vi "Deploy.vi"(6 "VI reference (current VI)":refnum<vi>, 8 "error in (no error)":errorcluster, 9 "Network Settings in":T3, 10 "Targets in":T4 {"Filtered Targets"."IP Mode" items=["Static"=1, "DHCP/Link-Local"=2, "Link-Local Only"=4, "DHCP Only"=8]}, 11 "Ctl Refs in":T7) -> (0 "error out":errorcluster, 1 "Network Settings out":T3, 2 "Targets out":T4 {"Filtered Targets"."IP Mode" items=["Static"=1, "DHCP/Link-Local"=2, "Link-Local Only"=4, "DHCP Only"=8]}, 3 "Ctl Refs out":T7, 4 "Button State":T2, 5 "Execution State":T1)   [LabVIEW 2013]
uses:
  Controls/Refs.ctl
  Controls/Button Refs.ctl
  Controls/Tab Ctl Refs.ctl
  types/TabStateType.ctl
  Controls/Indicator Refs.ctl
  Controls/Slider Refs.ctl
  Controls/Control Refs.ctl
  Controls/Targets.ctl
  Controls/Detected.ctl
  types/MAX Sys Cfg Target Information.ctl
  Controls/Network Settings.ctl
  types/ButtonStateType.ctl
  types/ExecutionStateType.ctl
  globals/Globals.vi
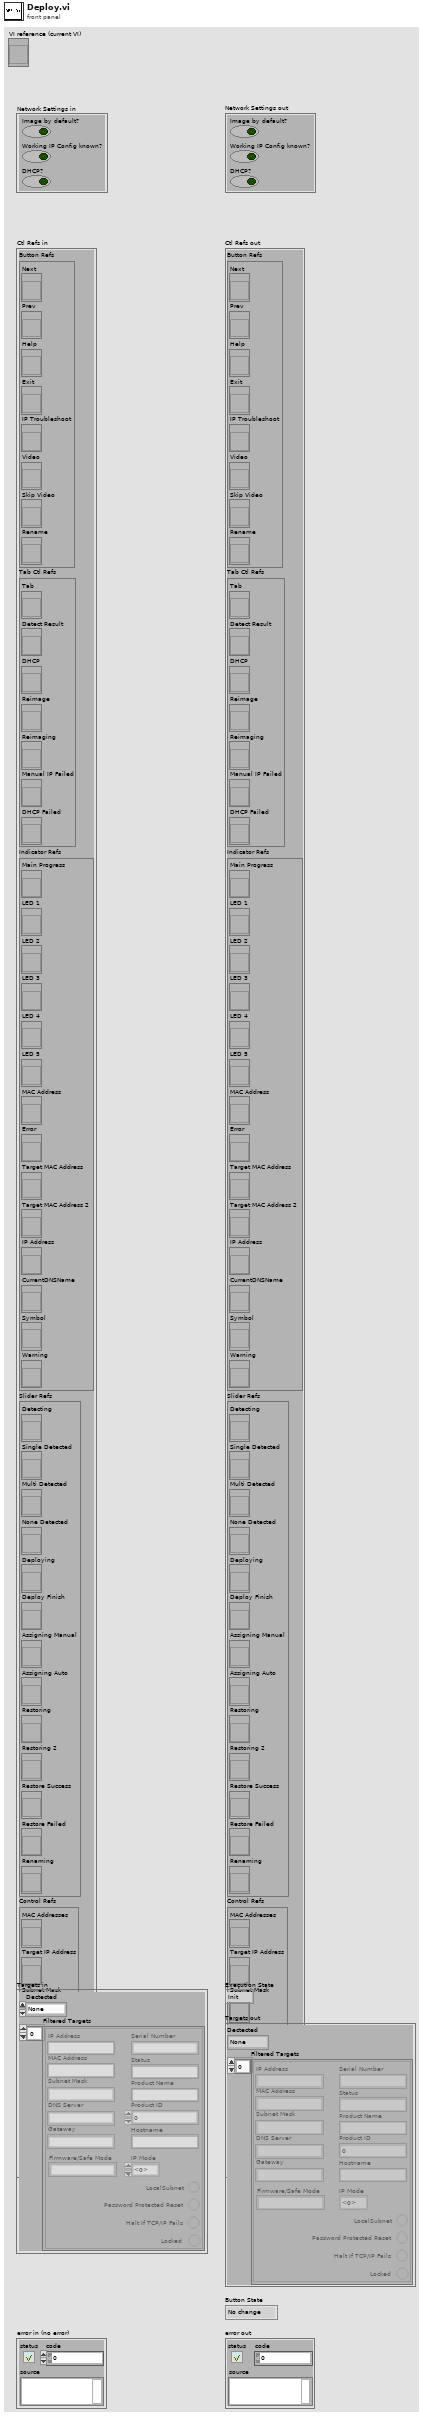
[diagram p1: front panel]
types:
  T1 = typedef "ExecutionStateType.ctl" = enum16{"Init", "Welcome", "Idle", "Detect", "Run Detection", "Detect Fail", "Detect One", "Detect Mult", "Deploy", "DHCP", "Static IP", "Run Deployment", "Connect Verify", "Exit", "Video Wait", "Success", "Troubleshoot", "Troubleshoot 2", "RenameDNS"}
  T2 = typedef "ButtonStateType.ctl" = enum16{"No change", "No Next", "No Prev", "All Disabled", "All Enabled", "Exit Only"}
  T3 = typedef "Network Settings.ctl" = cluster{"Image by default?":bool, "Working IP Config known?":bool, "DHCP?":bool}
  T4 = typedef "Targets.ctl" = cluster{"Dectected":T5, "Filtered Targets":T6[]}
  T5 = typedef "Detected.ctl" = enum16{"None", "Failed", "Single", "Multi"}
  T6 = typedef "MAX Sys Cfg Target Information.ctl" = cluster{"MAC Address":string, "IP Address":string, "Status":string, "Product Name":string, "Hostname":string, "Firmware/Safe Mode":string, "Subnet Mask":string, "Gateway":string, "DNS Server":string, "Serial Number":string, "Product ID":u32, "Locked ":bool, "LocalSubnet":bool, "Halt If TCP/IP Fails":bool, "Password Protected Reset":bool, "IP Mode":i32}
  T7 = typedef "Refs.ctl" = cluster{"Button Refs":T8, "Tab Ctl Refs":T9, "Indicator Refs":T10, "Slider Refs":T11, "Control Refs":T12, "Deploy Message":refnum<vi>}
  T8 = typedef "Button Refs.ctl" = cluster{"Next":refnum<vi>, "Prev":refnum<vi>, "Help":refnum<vi>, "Exit":refnum<vi>, "IP Troubleshoot":refnum<vi>, "Video":refnum<vi>, "Skip Video":refnum<vi>, "Rename":refnum<vi>}
  T9 = typedef "Tab Ctl Refs.ctl" = cluster{"Tab":refnum<vi>, "Detect Result":refnum<vi>, "DHCP":refnum<vi>, "Reimage":refnum<vi>, "Reimaging":refnum<vi>, "Manual IP Failed":refnum<vi>, "DHCP Failed":refnum<vi>}
  T10 = typedef "Indicator Refs.ctl" = cluster{"Main Progress":refnum<vi>, "LED 1":refnum<vi>, "LED 2":refnum<vi>, "LED 3":refnum<vi>, "LED 4":refnum<vi>, "LED 5":refnum<vi>, "MAC Address":refnum<vi>, "Error":refnum<vi>, "Target MAC Address":refnum<vi>, "Target MAC Address 2":refnum<vi>, "IP Address":refnum<vi>, "CurrentDNSName":refnum<vi>, "Symbol":refnum<vi>, "Warning":refnum<vi>}
  T11 = typedef "Slider Refs.ctl" = cluster{"Detecting":refnum<vi>, "Single Detected":refnum<vi>, "Multi Detected":refnum<vi>, "None Detected":refnum<vi>, "Deploying":refnum<vi>, "Deploy Finish":refnum<vi>, "Assigning Manual":refnum<vi>, "Assigning Auto":refnum<vi>, "Restoring":refnum<vi>, "Restoring 2":refnum<vi>, "Restore Success":refnum<vi>, "Restore Failed":refnum<vi>, "Renaming":refnum<vi>}
  T12 = typedef "Control Refs.ctl" = cluster{"MAC Addresses":refnum<vi>, "Target IP Address":refnum<vi>, "Subnet Mask":refnum<vi>, "DNS IP":refnum<vi>, "Default Gateway":refnum<vi>, "DNSName":refnum<vi>}
  T13 = enum32{"Welcome", "Instructions", "Detect", "Run Detection", "Detect Result", "Deploy", "Run Deployment", "Connect Verify", "Success", "DHCP", "Troubleshoot", "System Restore"}
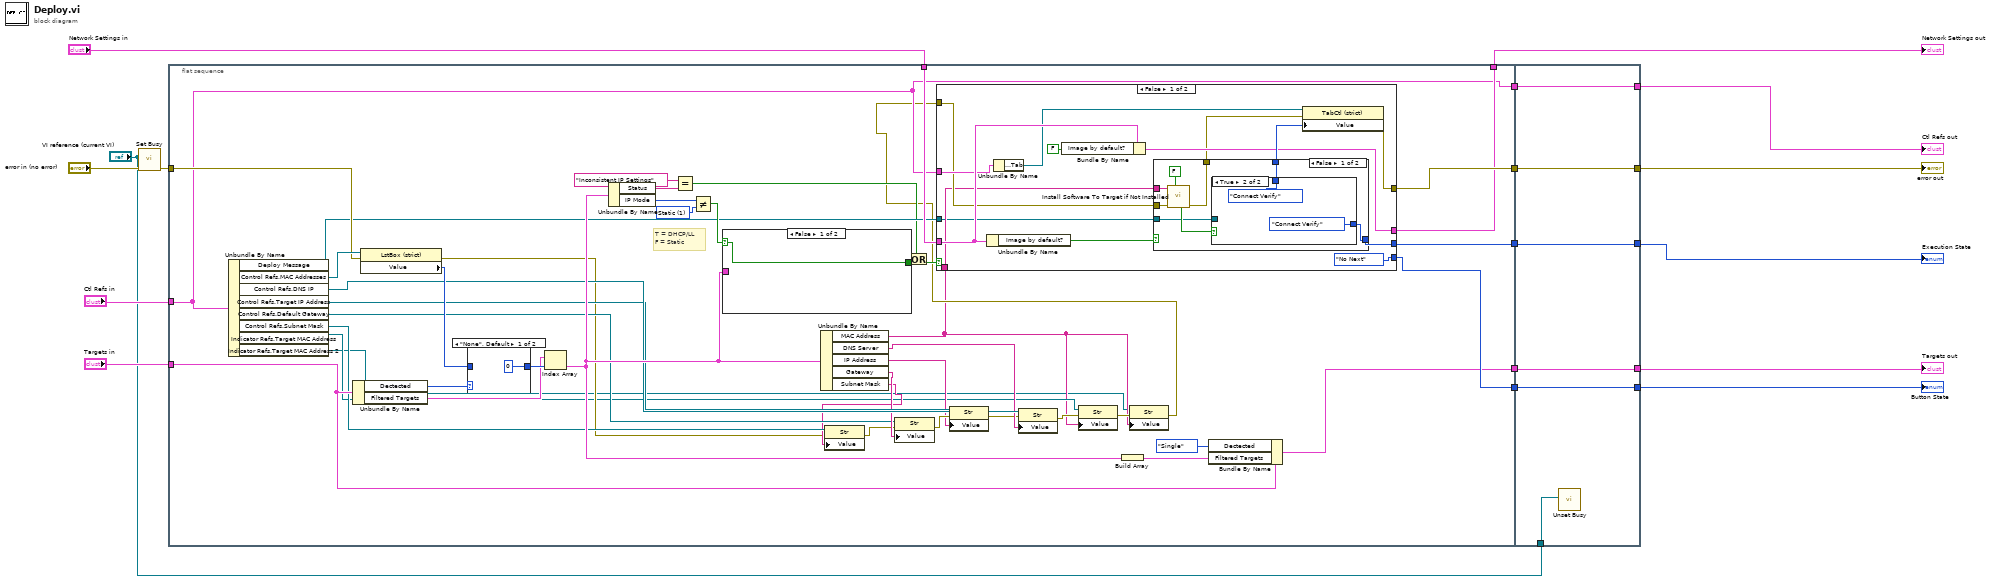
[diagram p0: block diagram]
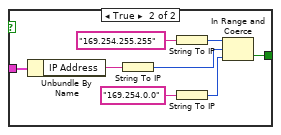
[diagram p2: hidden frame]
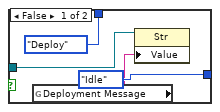
[diagram p3: hidden frame]
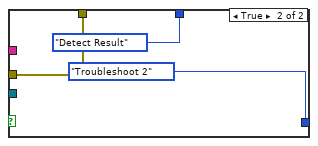
[diagram p4: hidden frame]
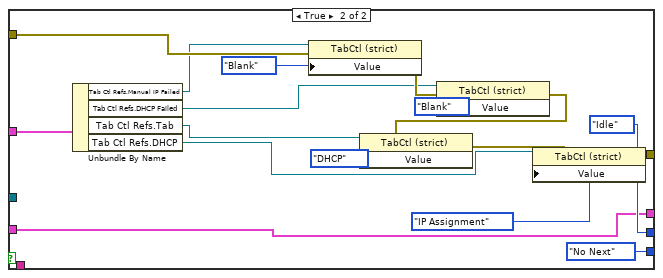
[diagram p5: hidden frame]
diagram:
  n1 = call <vilib>:"Set Busy.vi"("error in (no error)"="error in (no error)", "VI reference (current VI)"="VI reference (current VI)") -> ("error out"=w7:errorcluster)  [unwired: 8 in, 1 out]
  n2 = flat-sequence {
    tunnel: "Network Settings in" -> [w57]
    tunnel: [w56] -> w12
    tunnel: "Targets in" -> [w49]
    tunnel: "Ctl Refs in" -> [w31]
    tunnel: w7 -> [w44]
    tunnel: [w60] -> w6
    tunnel: [w59] -> w5
    tunnel: [w58] -> w4
    tunnel: [w46] -> w3
    tunnel: [w31] -> w2
    tunnel: [w122] -> w17
    tunnel: [w123] -> w14
    tunnel: [w124] -> w10
    tunnel: [w125] -> w9
    tunnel: [w126] -> w8
    tunnel: w6 -> [w126]
    tunnel: w5 -> [w125]
    tunnel: w4 -> [w124]
    tunnel: w3 -> [w123]
    tunnel: w2 -> [w122]
    tunnel: "VI reference (current VI)" -> [w121]
    frame #0 {
      w27 = 1 items=["Static"=1, "DHCP/Link-Local"=2, "Link-Local Only"=4, "DHCP Only"=8] ("Primary NIC:IP Address Request Mode")
      # "T = DHCP/LL\nF = Static"
      n3 = Unbundle By Name(w31) -> ("Deploy Message"=w28:refnum<vi>, "Control Refs.MAC Addresses"=w45:refnum<vi>, "Control Refs.DNS IP"=w42:refnum<vi>, "Control Refs.Target IP Address"=w40:refnum<vi>, "Control Refs.Default Gateway"=w38:refnum<vi>, "Control Refs.Subnet Mask"=w37:refnum<vi>, "Indicator Refs.Target MAC Address"=w22:refnum<vi>, "Indicator Refs.Target MAC Address 2"=w18:refnum<vi>)
      n4 = Unbundle By Name(w49) -> ("Dectected"=w50:T5, "Filtered Targets"=w51:T6[])
      n5 = property class="LstBox (strict)"(reference=w45, error in=w44) -> (error out=w32:errorcluster, "Value"=w43:i32)  [unwired: 1 out]
      n6 = case shown="\"None\", Default" w50 {
        tunnel: w43 -> [_ w120]
        tunnel: [0 w120] -> w61
        frame "None", Default {
        }
        frame "Multi" {
        }
      }
      n7 = Index Array(array=w51, index=w61) -> (element=w52:T6)
      n8 = Unbundle By Name(w52) -> ("Status"=w26:string, "IP Mode"=w54:i32)
      n9 = Equal?(x="Inconsistent IP Settings", y=w26) -> (x = y?=w23:bool)
      n10 = Not Equal?(x=w54, y=w27) -> (x != y?=w53:bool)
      n11 = case shown="False" w53 {
        selector: w53 -> [w62 _]
        tunnel: [w62 w65] -> w55
        tunnel: w52 -> [_ w63]
        frame False {
        }
        frame True {
          n12 = Unbundle By Name(w63) -> ("IP Address"=w64:string)
          n13 = String To IP(1:w64) -> (0:w66:u32)
          n14 = String To IP(1:"169.254.255.255" ("name")) -> (0:w68:u32)
          n15 = String To IP(1:"169.254.0.0" ("name")) -> (0:w67:u32)
          n16 = In Range and Coerce(upper limit=w68, x=w66, lower limit=w67) -> (In Range?=w65:bool)  [unwired: 1 out]
        }
      }
      n17 = Unbundle By Name(w52) -> ("MAC Address"=w19:string, "DNS Server"=w41:string, "IP Address"=w29:string, "Gateway"=w39:string, "Subnet Mask"=w36:string)
      n18 = property class="Str"(reference=w37, error in=w32, "Value"=w36) -> (error out=w35:errorcluster)  [unwired: 1 out]
      n19 = property class="Str"(reference=w38, error in=w35, "Value"=w39) -> (error out=w34:errorcluster)  [unwired: 1 out]
      n20 = Or(x=w23, y=w55) -> (x .or. y?=w24:bool)
      n21 = property class="Str"(reference=w40, error in=w34, "Value"=w29) -> (error out=w33:errorcluster)  [unwired: 1 out]
      n22 = property class="Str"(reference=w42, error in=w33, "Value"=w41) -> (error out=w30:errorcluster)  [unwired: 1 out]
      n23 = property class="Str"(reference=w22, error in=w30, "Value"=w19) -> (error out=w21:errorcluster)  [unwired: 1 out]
      n24 = Build Array(w52) -> (w47:T6[])
      n25 = property class="Str"(reference=w18, error in=w21, "Value"=w19) -> (error out=w20:errorcluster)  [unwired: 1 out]
      n26 = case shown="False" w24 {
        tunnel: w20 -> [w74 w114]
        tunnel: [w84 w117] -> w60
        tunnel: [w82 ExecutionStateType."Idle" ("Enum")] -> w59
        tunnel: [ButtonStateType."No Next" ("Enum") ButtonStateType."No Next" ("Enum")] -> w58
        tunnel: w57 -> [w80 w107]
        tunnel: [w77 w107] -> w56
        tunnel: w31 -> [w76 w106]
        tunnel: w19 -> [w73 _]
        tunnel: w28 -> [w71 _]
        frame False {
          n27 = Unbundle By Name(w80) -> ("Image by default?"=w78:bool)
          n28 = Unbundle By Name(w76) -> ("Tab Ctl Refs.Tab"=w75:refnum<vi>)
          n29 = Bundle By Name(cluster=w80, "Image by default?"=FALSE) -> (w77:T3)
          n30 = case shown="False" w78 {
            tunnel: [w92 ExecutionStateType."Troubleshoot 2" ("Enum")] -> w82
            tunnel: [w91 T13."Detect Result" ("Tab Control")] -> w81
            tunnel: w74 -> [w90 w99]
            tunnel: w73 -> [w89 _]
            tunnel: [w87 w99] -> w72
            tunnel: w71 -> [w85 _]
            frame False {
              n31 = call "Install Software To Target if Not Installed.vi"("Install (T)"=FALSE, "error in (no error)"=w90, "MAC Address"=w89) -> ("error out"=w87:errorcluster, "Installed"=w86:bool)  [unwired: 7 in]
              n32 = case shown="True" w86 {
                tunnel: [ExecutionStateType."Idle" ("Enum") ExecutionStateType."Connect Verify" ("Enum")] -> w92
                tunnel: [T13."Deploy" ("Tab Control") T13."Connect Verify" ("Tab Control")] -> w91
                tunnel: w85 -> [w94 _]
                frame False {
                  n33 = global read "Globals.vi" "Deployment Message"() -> (w93:string)
                  n34 = property class="Str"(reference=w94, "Value"=w93) -> ()  [unwired: 1 in, 2 out]
                }
                frame True {
                }
              }
            }
            frame True {
            }
          }
          n35 = property on="Property Node" class="TabCtl (strict)"(reference=w75, error in=w72, "Value"=w81) -> (error out=w84:errorcluster)  [unwired: 1 out]
        }
        frame True {
          n36 = Unbundle By Name(w106) -> ("Tab Ctl Refs.Manual IP Failed"=w105:refnum<vi>, "Tab Ctl Refs.DHCP Failed"=w104:refnum<vi>, "Tab Ctl Refs.Tab"=w103:refnum<vi>, "Tab Ctl Refs.DHCP"=w102:refnum<vi>)
          n37 = property on="Property Node" class="TabCtl (strict)"(reference=w105, error in=w114, "Value"=enum32{"Failed", "Blank"}."Blank" ("Manual IP Failed Tab")) -> (error out=w113:errorcluster)  [unwired: 1 out]
          n38 = property on="Property Node" class="TabCtl (strict)"(reference=w104, error in=w113, "Value"=enum32{"Failed", "Blank"}."Blank" ("DHCP Failed Tab")) -> (error out=w112:errorcluster)  [unwired: 1 out]
          n39 = property on="Property Node" class="TabCtl (strict)"(reference=w103, error in=w112, "Value"=T13."DHCP" ("Tab Control")) -> (error out=w118:errorcluster)  [unwired: 1 out]
          n40 = property on="Property Node" class="TabCtl (strict)"(reference=w102, error in=w118, "Value"=enum32{"IP Assignment", "DHCP", "Manual IP"}."IP Assignment" ("DHCP Tabs")) -> (error out=w117:errorcluster)  [unwired: 1 out]
        }
      }
      n41 = Bundle By Name(cluster=w49, "Dectected"=Detected."Single", "Filtered Targets"=w47) -> (w46:T4)
    }
    frame #1 {
      n42 = call <vilib>:"Unset Busy.vi"("VI reference (current VI)"=w121) -> ()  [unwired: 10 in, 1 out]
    }
  }
  "Ctl Refs out" <- w17
  "Targets out" <- w14
  "Network Settings out" <- w12
  "Button State" <- w10
  "Execution State" <- w9
  "error out" <- w8
